vi "load default verify paths.vi"(8 "error in":errorcluster, 11 "connection creator in":refnum<class "connection creator.lvclass">) -> (0 "error out":errorcluster)   [LabVIEW 2016, in "connection creator.lvclass"]
uses:
  connection creator.lvclass
  connection creator.lvclass/connection creator.ctl
  dllwrapper/async tls dl.lvlib
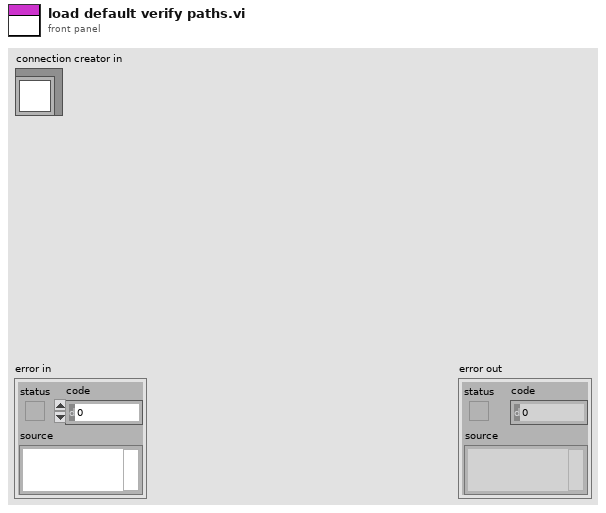
[diagram p1: front panel]
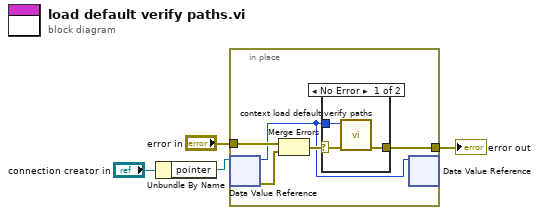
[diagram p0: block diagram]
diagram:
  n1 = Unbundle By Name("connection creator in") -> ("pointer"=w2:refnum<data-value>)
  n2 = in-place {
    in-place-border: "error in" -> [w8]
    in-place-border: [w6] -> w1
    n3 = in-place-dvr #1(w2) -> (w5:u64, w9:errorcluster)
    n4 = Merge Errors(w8, w9) -> (w7:errorcluster)
    n5 = case shown="No Error" w7 {
      selector: w7 -> [w12 w13]
      tunnel: [w10 w13] -> w6
      tunnel: w5 -> [w11 _]
      frame No Error {
        n6 = call "context load default verify paths.vi"("error in"=w12, "connector"=w11) -> ("error out"=w10:errorcluster)  [unwired: 9 in]
      }
      frame Error {
      }
    }
    n7 = in-place-dvr #1(w5) -> ()  [unwired: 2 out]
  }
  "error out" <- w1
